vi "BRig_dataCurrent_L_ENL2_T_end_l2.vi"() -> (2 "output_L_ENL2_T_end_l2":i32)   [LabVIEW 2014]
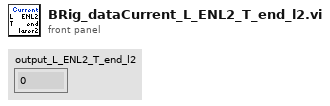
[diagram p1: front panel]
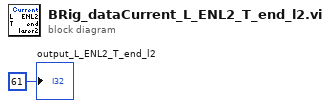
[diagram p0: block diagram]
diagram:
  "output_L_ENL2_T_end_l2" <- 61 ("output_iBlock")
